vi "string.vi"() -> ()   [LabVIEW 2020]
panel:
  out "date/time string":string
  out "resulting string":string
  out "output 1":dbl
  out "after substring":string
  out "match substring":string
  out "before substring":string
  out "result string":string
  out "substring":string
  out "concatenated string":string
  out "length":i32
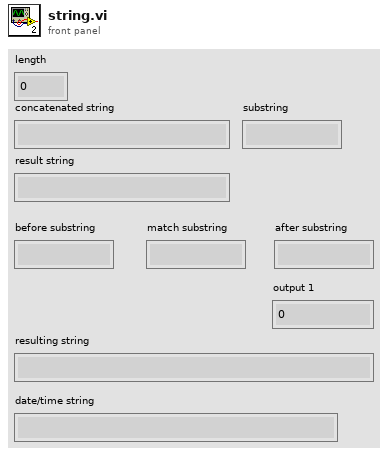
[diagram p1: front panel]
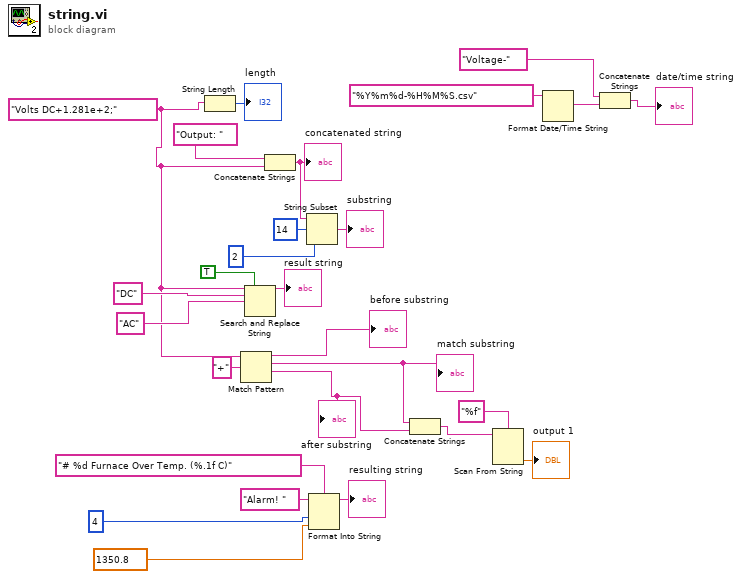
[diagram p0: block diagram]
diagram:
  w17 = "Volts DC+1.281e+2;"
  n1 = String Length(string=w17) -> (length=→"length":i32)
  n2 = Match Pattern(string=w17, regular expression="+") -> (before substring=→"before substring":string, match substring=w14:string, after substring=w13:string)  [unwired: 1 in, 1 out]
  "match substring" <- w14
  "after substring" <- w13
  n3 = Search and Replace String(replace all?=TRUE ("replace all? (F)"), input string=w17, search string="DC", replace string="AC" ("replace string (\"\")")) -> (result string=→"result string":string)  [unwired: 4 in, 3 out]
  n4 = Concatenate Strings("Output: " ("string"), w17) -> (w25:string)
  "concatenated string" <- w25
  n5 = String Subset(string=w25, offset (0)=14, length (rest)=2 ("length (rest)")) -> (substring=→"substring":string)
  n6 = Format Into String(format string="# %d Furnace Over Temp. (%.1f C)", initial string="Alarm! ", 4, 1350.8) -> (resulting string=→"resulting string":string)  [unwired: 1 in, 1 out]
  n7 = Concatenate Strings(w14, w13) -> (w12:string)
  n8 = Scan From String(format string="%f", input string=w12) -> (output 1=→"output 1":dbl)  [unwired: 3 in, 3 out]
  n9 = Format Date/Time String(time format string (%c)="%Y%m%d-%H%M%S.csv") -> (date/time string=w2:string)  [unwired: 2 in]
  n10 = Concatenate Strings("Voltage-", w2) -> (→"date/time string":string)
